vi "Startup.vi"(6 "LabVIEW Web Service":refnum<class "Web Service.lvclass">) -> ()   [LabVIEW 2015]
uses:
  <vilib>/wsapi/Web Service.lvclass
  Classes/Server/JSONRPC Server.lvclass
panel:
  # "Use the web service input terminal to call the VIs on the Service subpalette of the Web Services palette. Do not remove it from the connector pane unless you don't need access to the palette."
  # "Any additional terminals added to the connector pane of a startup VI will be ignored."
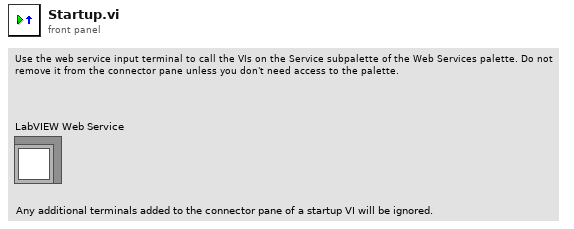
[diagram p1: front panel]
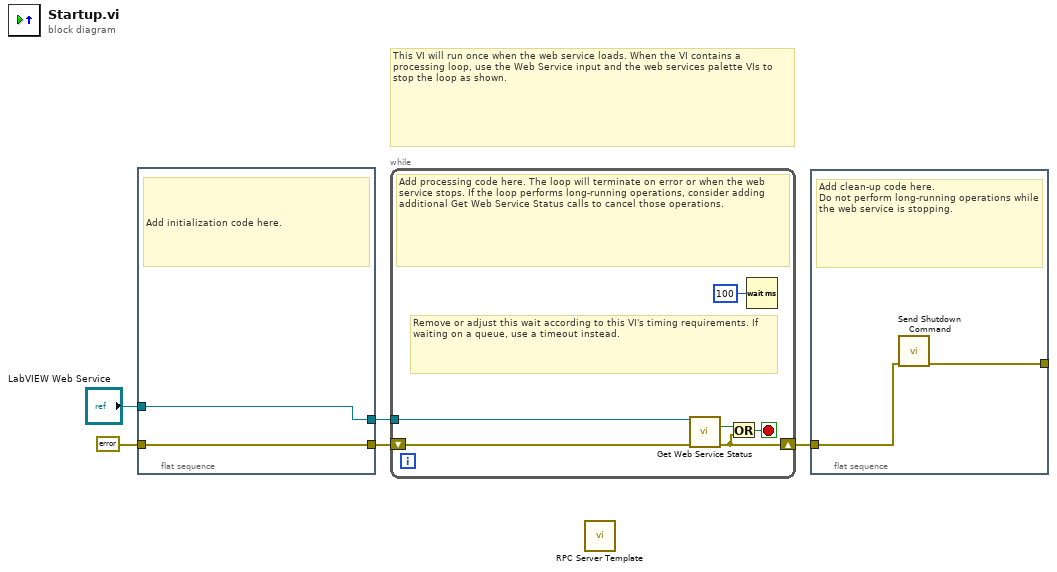
[diagram p0: block diagram]
diagram:
  # "This VI will run once when the web service loads. When the VI contains a processing loop, use the Web Service input and the web services palette VIs to stop the loop as shown."
  n1 = flat-sequence {
    tunnel: "LabVIEW Web Service" -> [w7]
    tunnel: [w7] -> w4
    tunnel: [w6] -> w3
    tunnel: errorcluster {"status"=FALSE, "code"=0, "source"=""} ("error constant") -> [w6]
    frame #0 {
      # "Add initialization code here."
    }
  }
  n2 = while {
    tunnel: w4 -> [w12]
    shift-right: [w9] -> w1
    shift-left: w3 -> [w10]
    stop <- w11 stop-if-true
    # "Remove or adjust this wait according to this VI's timing requirements. If waiting on a queue, use a timeout instead."
    # "Add processing code here. The loop will terminate on error or when the web service stops. If the loop performs long-running operations, consider adding additional Get Web Service Status calls to cancel those operations."
    n3 = call <vilib>:"Get Web Service Status.vi"("LabVIEW Web Service"=w12, "error in (no error)"=w10) -> ("service stopping?"=w13:bool, "error out"=w9:errorcluster)  [unwired: 11 in, 1 out]
    n4 = Or(x=w13, y=w9) -> (x .or. y?=w11:bool)
    n5 = Wait (ms)(milliseconds to wait=u32 100) -> ()  [unwired: 1 out]
  }
  n6 = call "RPC Server Template.vi"() -> ()  [unwired: 11 in, 1 out]
  n7 = flat-sequence {
    tunnel: w1 -> [w15]
    tunnel: [w14] -> _
    frame #0 {
      # "Add clean-up code here.\nDo not perform long-running operations while the web service is stopping."
      n8 = call "Send Shutdown Command.vi"("error in (no error)"=w15) -> ("error out"=w14:errorcluster)  [unwired: 10 in]
    }
  }
